vi "Example_MCA_Program.vi"() -> ()   [LabVIEW 2014]
uses:
  Typedef_MCAControl.ctl
panel:
  in  "TAC Settings":cluster{"Full Scale (ns)":dbl, "# bins":i32}={"Full Scale (ns)"=1000.0, "# bins"=1000} {"# bins" min=1 max=65535 step=1; "Full Scale (ns)" format="%0.2f"}
  in  "Reset":bool
  in  "Pause":bool
  out "Coincidence Signal":cluster{"Axis":dbl[], i32[]}(graph)
  out "Total Time (s)":dbl
  out "Delta Time (s)":dbl
  out "error out":errorcluster
  in  "Update Rate (Hz)":u32=10 min=1 max=1000 step=1
  in  "Stop Button":bool
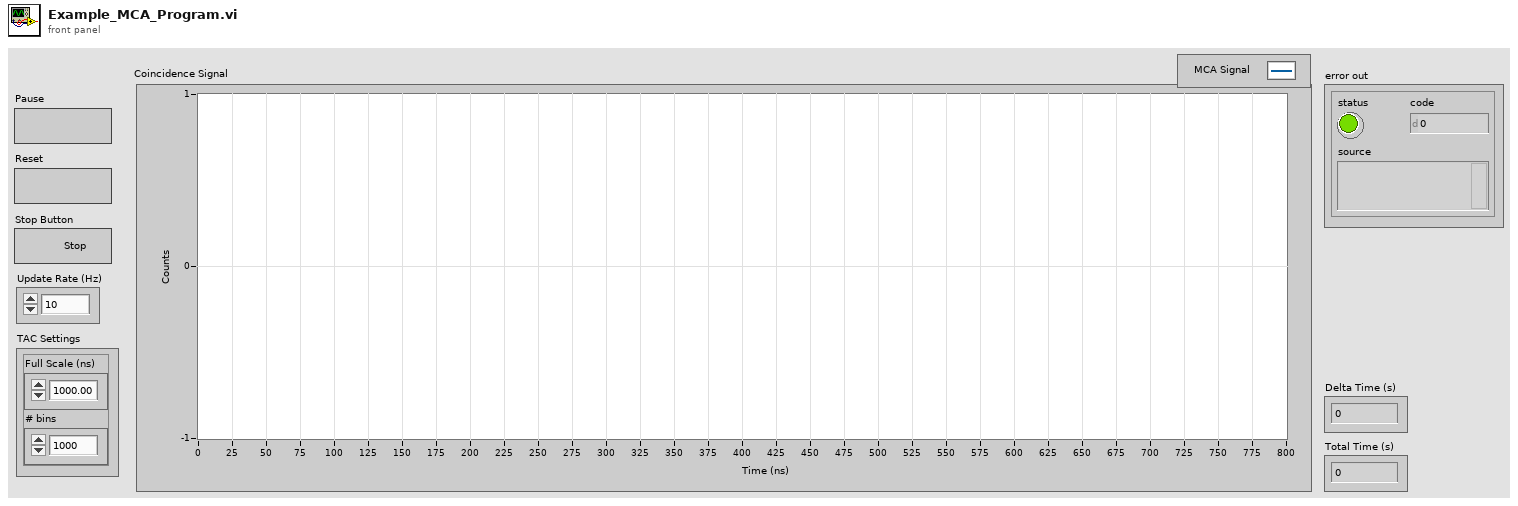
[diagram p1: front panel]
types:
  T1 = enum16{"Start Running", "Stop Running", "Check State"}
  T2 = typedef "Typedef_MCAControl.ctl" = enum16{"Start", "Check", "Pause", "Unpause", "Update Settings", "Reset", "Stop"}
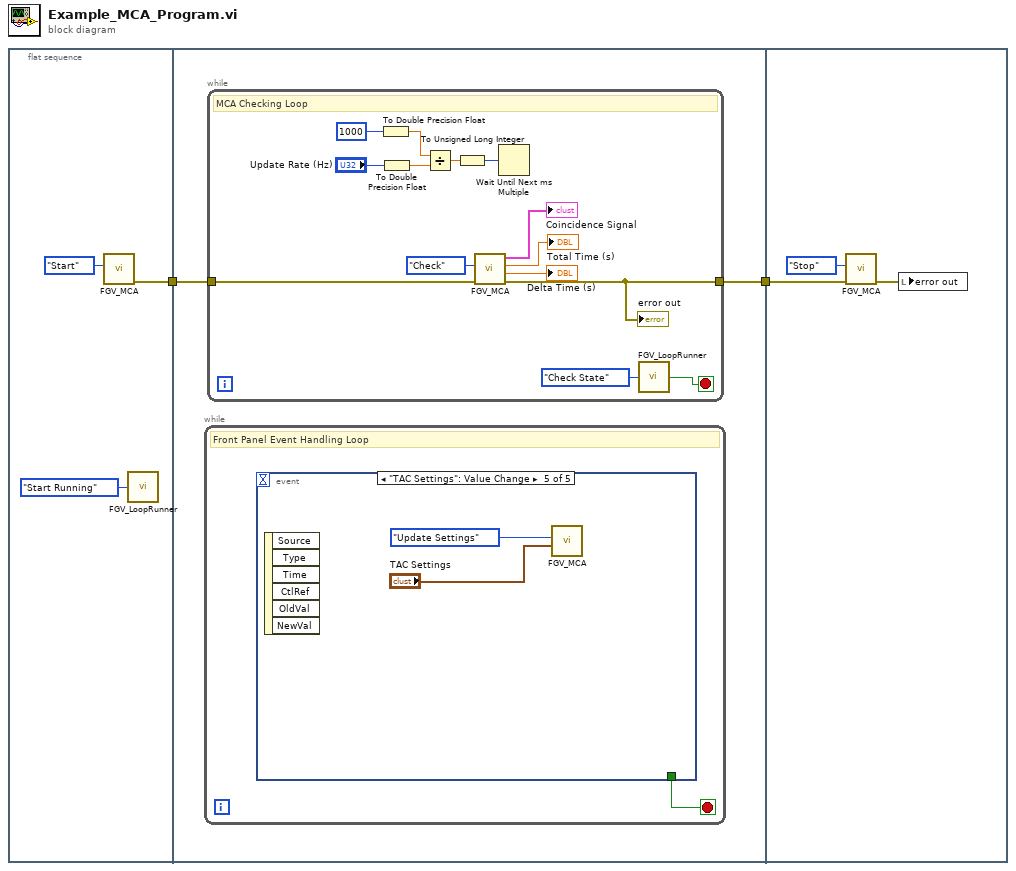
[diagram p0: block diagram]
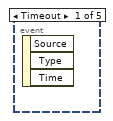
[diagram p2: hidden frame]
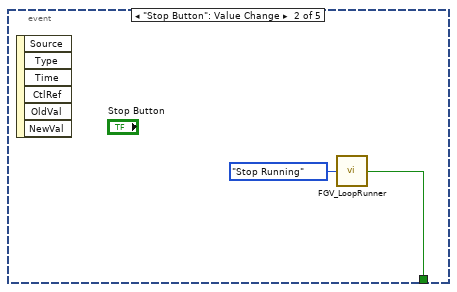
[diagram p3: hidden frame]
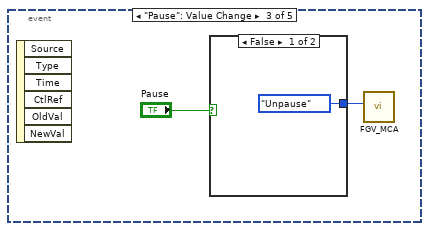
[diagram p4: hidden frame]
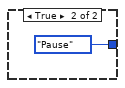
[diagram p5: hidden frame]
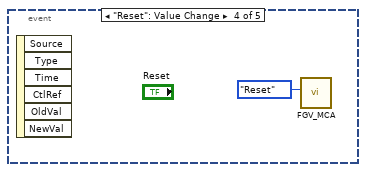
[diagram p6: hidden frame]
diagram:
  n1 = flat-sequence {
    tunnel: [w3] -> w2
    tunnel: w2 -> [w7]
    tunnel: [w6] -> w1
    tunnel: w1 -> [w33]
    frame #0 {
      n2 = call "FGV_MCA.vi"("MCA Action"=Typedef_MCAControl."Start") -> ("error out"=w3:errorcluster)  [unwired: 6 in, 4 out]
      n3 = call "FGV_LoopRunner.vi"("Loop Controller"=T1."Start Running") -> ()  [unwired: 1 out]
    }
    frame #1 {
      n4 = while {
        stop <- w22 stop-if-true
        # "Front Panel Event Handling Loop"
        n5 = event shown="[4] \"TAC Settings\": Value Change" {
          selector: _ -> [_ _ _ _ _]
          dyn-events: _ -> [_ _ _ _ _]
          timeout: _ -> [_ _ _ _ _]
          tunnel: [_ w23 _ _ _] -> w22
          event Timeout {
            n6 = event-data() -> ()  [unwired: 1 in, 3 out]
          }
          event "Stop Button": Value Change {
            n7 = event-data() -> ()  [unwired: 1 in, 6 out]
            n8 = call "FGV_LoopRunner.vi"("Loop Controller"=T1."Stop Running") -> ("Stop Loops"=w23:bool)
          }
          event "Pause": Value Change {
            n9 = event-data() -> ()  [unwired: 1 in, 6 out]
            n10 = case shown="False" "Pause" {
              tunnel: [Typedef_MCAControl."Unpause" ("MCA Action") Typedef_MCAControl."Pause" ("MCA Action")] -> w25
              frame False {
              }
              frame True {
              }
            }
            n11 = call "FGV_MCA.vi"("MCA Action"=w25) -> ()  [unwired: 6 in, 5 out]
          }
          event "Reset": Value Change {
            n12 = event-data() -> ()  [unwired: 1 in, 6 out]
            n13 = call "FGV_MCA.vi"("MCA Action"=Typedef_MCAControl."Reset") -> ()  [unwired: 6 in, 5 out]
          }
          event "TAC Settings": Value Change {
            n14 = event-data() -> ()  [unwired: 1 in, 6 out]
            n15 = call "FGV_MCA.vi"("TAC Settings"="TAC Settings", "MCA Action"=Typedef_MCAControl."Update Settings") -> ()  [unwired: 5 in, 5 out]
          }
        }
      }
      n16 = while {
        tunnel: w7 -> [w12]
        tunnel: [w11] -> w6
        stop <- w21 stop-if-true
        # "MCA Checking Loop"
        n17 = To Double Precision Float(number=u32 1000 ("x")) -> (double precision float=w13:dbl)
        n18 = To Double Precision Float(number="Update Rate (Hz)") -> (double precision float=w14:dbl)
        n19 = Divide(x=w13, y=w14) -> (x/y=w16:dbl)
        n20 = To Unsigned Long Integer(number=w16) -> (unsigned 32bit integer=w15:u32)
        n21 = call "FGV_MCA.vi"("Error In"=w12, "MCA Action"=Typedef_MCAControl."Check") -> ("error out"=w11:errorcluster, "Delta Time (s)"=→"Delta Time (s)":dbl, "Total Time (s)"=→"Total Time (s)":dbl, "Coincidence Signal"=→"Coincidence Signal":cluster{"Axis":dbl[], i32[]})  [unwired: 5 in, 1 out]
        "error out" <- w11
        n22 = Wait Until Next ms Multiple(millisecond multiple=w15) -> ()  [unwired: 1 out]
        n23 = call "FGV_LoopRunner.vi"("Loop Controller"=T1."Check State") -> ("Stop Loops"=w21:bool)
      }
    }
    frame #2 {
      n24 = call "FGV_MCA.vi"("Error In"=w33, "MCA Action"=Typedef_MCAControl."Stop") -> ("error out"=w32:errorcluster)  [unwired: 5 in, 4 out]
      n25 = local write "error out"(w32) -> ()
    }
  }
